vi "PXI-4132 Init Channel (RT).vi"(5 "Channel Type":T3 items=["Voltage Controlled", "Current Controlled"], 7 "Channel Sense":T2=1008 items=["Local"=1008, "Remote"=1009], 8 "error in (no error)":errorcluster, 10 "resource name":refnum<k15>="Dev1", 11 "Device Reference In":T1 format="%.0x") -> (0 "error out":errorcluster, 2 "resource name Out":refnum<k15>="Dev1", 3 "Device Reference Out":T1 format="%.0x", 4 "Defaults":dbl[](array[numeric]), 6 "FIFO Indexes":i32[](array[numeric]))   [LabVIEW 2013, in "PXI-4132 Custom Device.lvlib"]
uses:
  PXI-4132 Custom Device.lvlib
  Channel Type.ctl
  Channel Sense.ctl
  <vilib>/NI Veristand/Custom Device API/Custom Device Item Ref.ctl
  <instrlib>/niDCPower/nidcpower.llb/niDCPower Output Function.ctl
  PXI-4132 Global Variable.vi
  <vilib>/NI Veristand/Custom Device Tools/Custom Device Utility Library/NI VeriStand - Search for Item by Property.vi
  <vilib>/NI Veristand/Custom Device Tools/Custom Device Utility Library/NI VeriStand - Search for Item by Name.vi
  <vilib>/NI VeriStand/Custom Device API/Custom Device API.lvlib
  <vilib>/NI Veristand/Custom Device Tools/Custom Device Utility Library/Custom Device Utility Library.lvlib
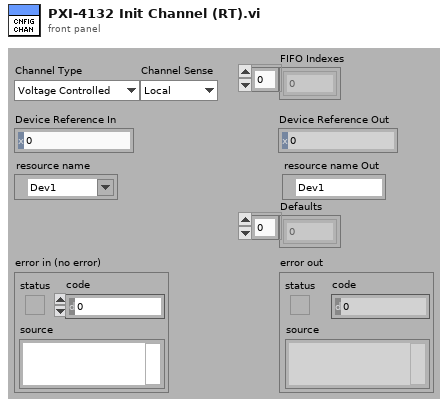
[diagram p1: front panel]
types:
  T1 = typedef "Custom Device API.lvlib/Custom Device Item Ref.ctl" = u64
  T2 = typedef "PXI-4132 Custom Device.lvlib/Channel Sense.ctl" = i32
  T3 = typedef "PXI-4132 Custom Device.lvlib/Channel Type.ctl" = i32
  T4 = typedef "Custom Device API.lvlib/Custom Device Channel.ctl" = cluster{"Type":T5, "Units":string, "Default Value":dbl, "Faultable":bool, "Scalable":bool}
  T5 = typedef "Custom Device API.lvlib/Custom Device Channel Type.ctl" = enum16{"Input", "Output"}
  T6 = typedef "niDCPower Output Function.ctl" = i32
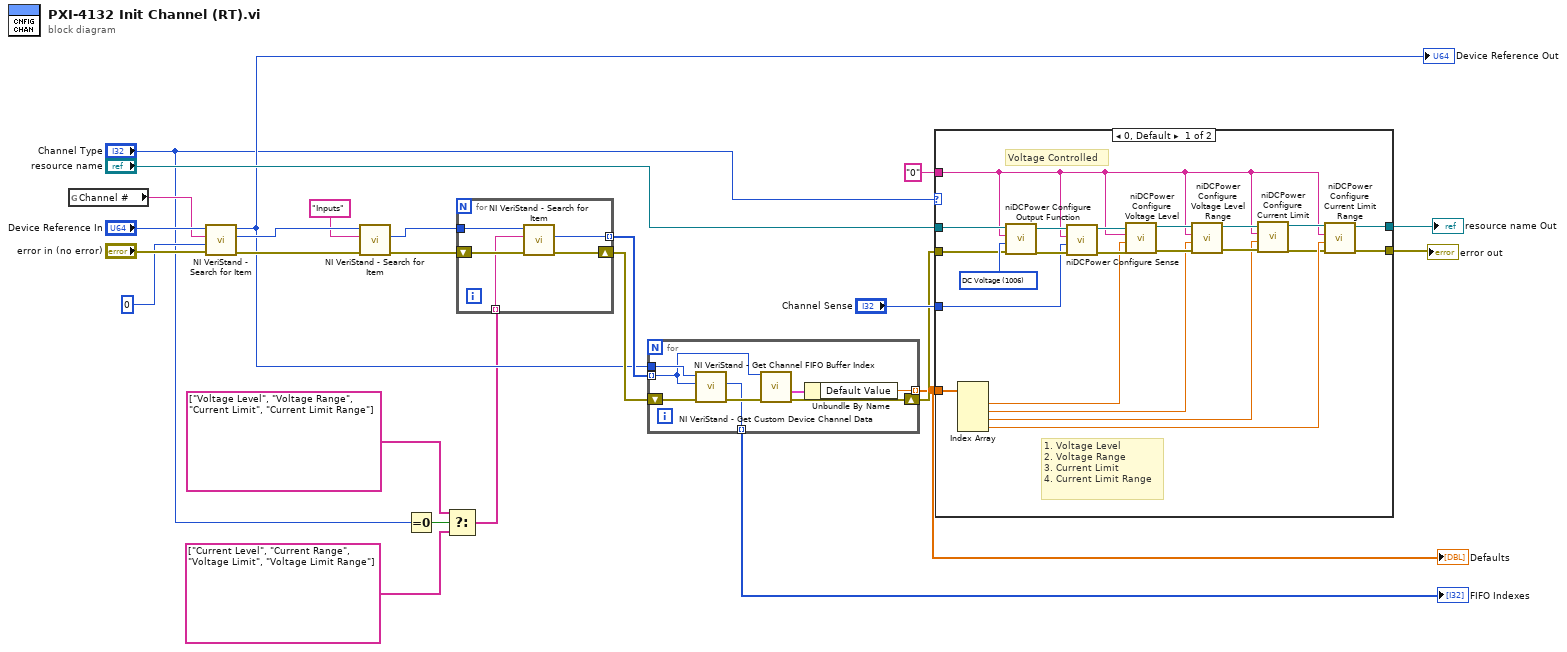
[diagram p0: block diagram]
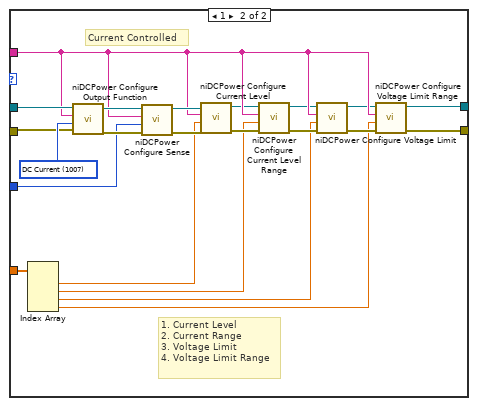
[diagram p2: hidden frame]
diagram:
  n1 = global read "PXI-4132 Global Variable.vi" "Channel #"() -> (w20:string)
  n2 = call-poly <vilib>:"NI VeriStand - Search for Item.vi"("error in"="error in (no error)", "Property Value"=0, "Property Name"=w20, "Section Ref in"="Device Reference In") -> ("error out"=w21:errorcluster, "Item Ref"=w18:T1, "Section Ref out"=w9:T1)  [unwired: 4 in, 1 out]
  "Device Reference Out" <- w9
  n3 = call-poly <vilib>:"NI VeriStand - Search for Item.vi"("error in"=w21, "Item Name"="Inputs" ("Channel Name"), "Section Ref in"=w18) -> ("error out"=w16:errorcluster, "Item Ref"=w12:T1)  [unwired: 5 in, 2 out]
  n4 = Equal To 0?(x="Channel Type") -> (x = 0?=w4:bool)
  n5 = Select(t=string[] ["Voltage Level", "Voltage Range", "Current Limit", "Current Limit Range"], s=w4, f=string[] ["Current Level", "Current Range", "Voltage Limit", "Voltage Limit Range"]) -> (s? t:f=w1:string[])
  n6 = for {
    tunnel: w12 -> [w29]
    tunnel: [w27] -> w10 mode=indexing
    shift-right: [w28] -> w11
    shift-left: w16 -> [w30]
    tunnel: w1 -> [w26] mode=indexing
    n7 = call-poly <vilib>:"NI VeriStand - Search for Item.vi"("error in"=w30, "Item Name"=w26, "Section Ref in"=w29) -> ("error out"=w28:errorcluster, "Item Ref"=w27:T1)  [unwired: 5 in, 2 out]
  }
  n8 = for {
    tunnel: w10 -> [w32] mode=indexing
    tunnel: [w37] -> w6 mode=indexing
    shift-right: [w35] -> w8
    shift-left: w11 -> [w36]
    tunnel: w9 -> [w33]
    tunnel: [w31] -> w7 mode=indexing
    n9 = call <vilib>:"NI VeriStand - Get Channel FIFO Buffer Index.vi"("error in"=w36, "Channel Ref"=w32, "Device Ref in"=w33) -> ("error out"=w34:errorcluster, "Channel FIFO Buffer Index"=w31:i32)  [unwired: 4 in, 3 out]
    n10 = call <vilib>:"NI VeriStand - Get Custom Device Channel Data.vi"("error in (no error)"=w34, "Channel Ref in"=w32) -> ("error out"=w35:errorcluster, "Channel"=w38:T4)  [unwired: 4 in, 4 out]
    n11 = Unbundle By Name(w38) -> ("Default Value"=w37:dbl)
  }
  "FIFO Indexes" <- w7
  "Defaults" <- w6
  n12 = case shown="0, Default" "Channel Type" {
    tunnel: w8 -> [w40 w62]
    tunnel: "resource name" -> [w57 w76]
    tunnel: "Channel Sense" -> [w54 w73]
    tunnel: [w53 w78] -> w23
    tunnel: [w52 w77] -> w24
    tunnel: "0" ("Channel Name") -> [w41 w74]
    tunnel: w6 -> [w39 w61]
    frame 0, Default {
      w60 = T6 1006 items=["DC Voltage"=1006, "DC Current"=1007] ("output function")
      # "1. Voltage Level\n2. Voltage Range\n3. Current Limit\n4. Current Limit Range"
      # "Voltage Controlled"
      n13 = Index Array(array=w39) -> (element #1=w51:dbl, element #2=w43:dbl, element #3=w42:dbl, element #4=w50:dbl)  [unwired: 4 in]
      n14 = call <instrlib>:"niDCPower Configure Output Function.vi"("error in (no error)"=w40, "output function"=w60, "channel name"=w41, "instrument handle"=w57) -> ("error out"=w58:errorcluster, "instrument handle out"=w59:refnum<k15>)  [unwired: 6 in]
      n15 = call <instrlib>:"niDCPower Configure Sense.vi"("error in (no error)"=w58, "sense"=w54, "channel name"=w41, "instrument handle"=w59) -> ("error out"=w56:errorcluster, "instrument handle out"=w55:refnum<k15>)  [unwired: 6 in]
      n16 = call <instrlib>:"niDCPower Configure Voltage Level.vi"("error in (no error)"=w56, "voltage level"=w51, "channel name"=w41, "instrument handle"=w55) -> ("error out"=w44:errorcluster, "instrument handle out"=w49:refnum<k15>)  [unwired: 6 in]
      n17 = call <instrlib>:"niDCPower Configure Voltage Level Range.vi"("error in (no error)"=w44, "voltage level range"=w43, "channel name"=w41, "instrument handle"=w49) -> ("error out"=w45:errorcluster, "instrument handle out"=w48:refnum<k15>)  [unwired: 6 in]
      n18 = call <instrlib>:"niDCPower Configure Current Limit.vi"("error in (no error)"=w45, "current limit"=w42, "channel name"=w41, "instrument handle"=w48) -> ("error out"=w46:errorcluster, "instrument handle out"=w47:refnum<k15>)  [unwired: 6 in]
      n19 = call <instrlib>:"niDCPower Configure Current Limit Range.vi"("error in (no error)"=w46, "current limit range"=w50, "channel name"=w41, "instrument handle"=w47) -> ("error out"=w52:errorcluster, "instrument handle out"=w53:refnum<k15>)  [unwired: 6 in]
    }
    frame 1 {
      w75 = T6 1007 items=["DC Voltage"=1006, "DC Current"=1007] ("output function")
      # "1. Current Level\n2. Current Range\n3. Voltage Limit\n4. Voltage Limit Range"
      # "Current Controlled"
      n20 = Index Array(array=w61) -> (element #1=w66:dbl, element #2=w65:dbl, element #3=w64:dbl, element #4=w63:dbl)  [unwired: 4 in]
      n21 = call <instrlib>:"niDCPower Configure Output Function.vi"("error in (no error)"=w62, "output function"=w75, "channel name"=w74, "instrument handle"=w76) -> ("error out"=w80:errorcluster, "instrument handle out"=w79:refnum<k15>)  [unwired: 6 in]
      n22 = call <instrlib>:"niDCPower Configure Sense.vi"("error in (no error)"=w80, "sense"=w73, "channel name"=w74, "instrument handle"=w79) -> ("error out"=w81:errorcluster, "instrument handle out"=w82:refnum<k15>)  [unwired: 6 in]
      n23 = call <instrlib>:"niDCPower Configure Current Level.vi"("error in (no error)"=w81, "current level"=w66, "channel name"=w74, "instrument handle"=w82) -> ("error out"=w67:errorcluster, "instrument handle out"=w68:refnum<k15>)  [unwired: 6 in]
      n24 = call <instrlib>:"niDCPower Configure Current Level Range.vi"("error in (no error)"=w67, "current level range"=w65, "channel name"=w74, "instrument handle"=w68) -> ("error out"=w69:errorcluster, "instrument handle out"=w72:refnum<k15>)  [unwired: 6 in]
      n25 = call <instrlib>:"niDCPower Configure Voltage Limit.vi"("error in (no error)"=w69, "voltage limit"=w64, "channel name"=w74, "instrument handle"=w72) -> ("error out"=w70:errorcluster, "instrument handle out"=w71:refnum<k15>)  [unwired: 6 in]
      n26 = call <instrlib>:"niDCPower Configure Voltage Limit Range.vi"("error in (no error)"=w70, "voltage limit range"=w63, "channel name"=w74, "instrument handle"=w71) -> ("error out"=w77:errorcluster, "instrument handle out"=w78:refnum<k15>)  [unwired: 6 in]
    }
  }
  "error out" <- w24
  "resource name Out" <- w23
